vi "rotate_point_by_radians_single.vi"(9 "theta":sgl, 10 "y":sgl, 11 "x":sgl) -> (2 "y out":sgl, 3 "x out":sgl)   [LabVIEW 2019]
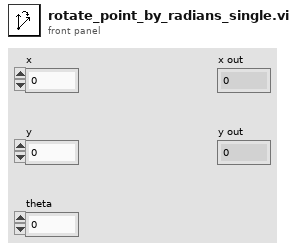
[diagram p1: front panel]
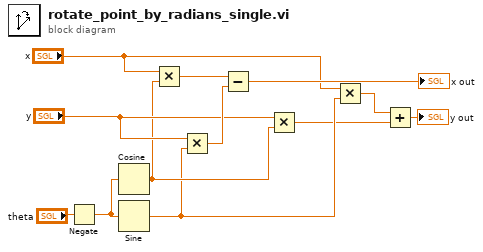
[diagram p0: block diagram]
diagram:
  n1 = Negate(x="theta") -> (-x=w1:sgl)
  n2 = Cosine(x=w1) -> (cos(x)=w9:sgl)
  n3 = Sine(x=w1) -> (sin(x)=w7:sgl)
  n4 = Multiply(x="x", y=w9) -> (x*y=w12:sgl)
  n5 = Multiply(x="y", y=w7) -> (x*y=w11:sgl)
  n6 = Subtract(x=w12, y=w11) -> (x-y=→"x out":sgl)
  n7 = Multiply(x="y", y=w9) -> (x*y=w5:sgl)
  n8 = Multiply(x="x", y=w7) -> (x*y=w6:sgl)
  n9 = Add(x=w6, y=w5) -> (x+y=→"y out":sgl)
